vi "NewDataInBuffer_Send.vi"(8 "error in (no error)":errorcluster, 9 "buffer location":u32, 10 "data group":string, 11 "Qbus in":refnum<class "Qbus.lvclass">) -> (0 "error out":errorcluster, 3 "Qbus out":refnum<class "Qbus.lvclass">)   [LabVIEW 2017, in "DataAccumulator.lvlib"]
uses:
  <vilib>/addons/InsightCM/Devices/Shared/Common/DataAccumulator/DataAccumulator.lvlib
  <vilib>/addons/Qbus/Qbus.lvclass
  <vilib>/addons/InsightCM/Devices/Shared/Common/DataAccumulator/controls/NewDataInBuffer.ctl
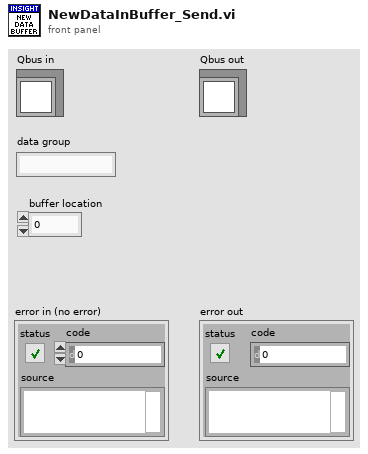
[diagram p1: front panel]
types:
  T1 = typedef "DataAccumulator.lvlib/NewDataInBuffer.ctl" = cluster{"DataGroup":string, "buffer location":u32}
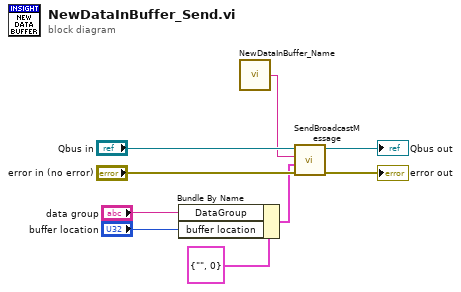
[diagram p0: block diagram]
diagram:
  n1 = Bundle By Name(cluster=T1 {"DataGroup"="", "buffer location"=0}, "DataGroup"="data group", "buffer location"="buffer location") -> (w2:T1)
  n2 = call <vilib>:"NewDataInBuffer_Name.vi"() -> ("MessageName"=w5:string)  [unwired: 5 in]
  n3 = call <vilib>:"SendBroadcastMessage.vi"("error in (no error)"="error in (no error)", "message value"=w2, "message name"=w5, "Qbus in"="Qbus in") -> ("error in (no error)"=→"error out":errorcluster, "Qbus out"=→"Qbus out":refnum<class "Qbus.lvclass">)  [unwired: 6 in]
